vi "CC Script Parse Define Random Dithering.vi"(8 "error in (no error)":errorcluster, 9 "To Script?":bool, 10 "Dithering Offsets in":T1, 11 "DefineDithering Parameters":string="\"Rnadome Dither Mispeller\" Count=3,Radius=1.23") -> (0 "error out":errorcluster, 1 "Name":string, 2 "Dithering Offsets out":T1, 3 "Script out":string="ObjectName \"RA\":\"123.456\",\"DEC\":\"4546.54\"")   [LabVIEW 2020]
uses:
  <vilib>/regexp/Match Regular Expression.xnode
  typedefs/CC Dithering Offsets.ctl
  typedefs/CC Dithering.ctl
  typedefs/CC cluster Offset Dithering.ctl
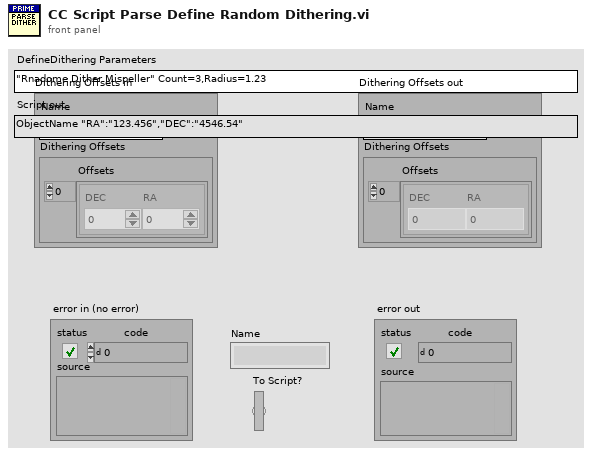
[diagram p1: front panel]
types:
  T1 = typedef "CC Dithering.ctl" = cluster{"Name":string, "Dithering Offsets":T2}
  T2 = typedef "CC cluster Offset Dithering.ctl" = cluster{"Offsets":T3[]}
  T3 = typedef "CC Dithering Offsets.ctl" = cluster{"DEC":dbl, "RA":dbl}
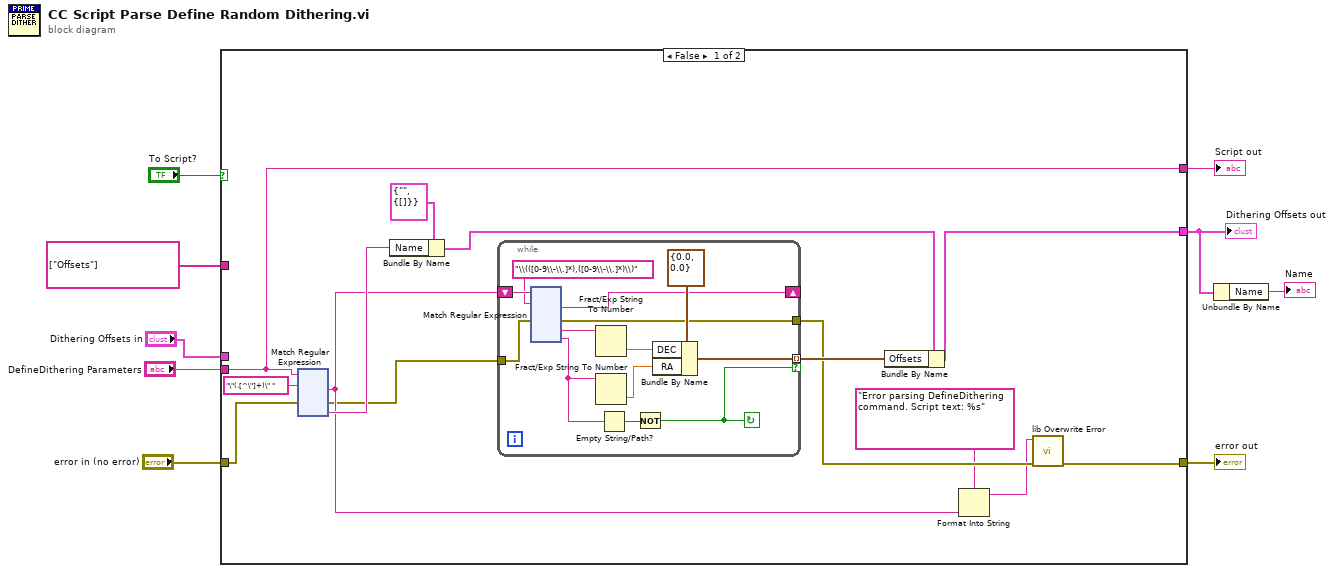
[diagram p0: block diagram]
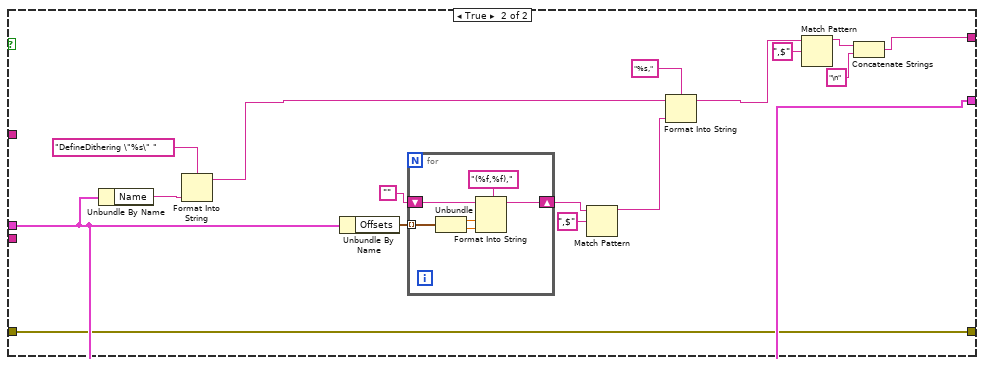
[diagram p2: hidden frame]
diagram:
  n1 = case shown="False" "To Script?" {
    tunnel: "DefineDithering Parameters" -> [w18 _]
    tunnel: string[] ["Offsets"] -> [_ _]
    tunnel: [w20 w278] -> w2
    tunnel: "error in (no error)" -> [w11 w276]
    tunnel: [w16 w276] -> w6
    tunnel: "Dithering Offsets in" -> [_ w278]
    tunnel: [w18 w277] -> w3
    frame False {
      n2 = xnode "Match Regular Expression"("input string"=w18, "regular expression"="\"(.[^\"]+)\" ", "error in"=w11) -> ("after match"=w13:string, "error out"=w10:errorcluster, "submatch 1"=w22:string)  [unwired: 3 in, 3 out]
      n3 = Bundle By Name(cluster=T1 {"Name"="", "Dithering Offsets"={"Offsets"=[]}} ("Dithering Offsets"), "Name"=w22) -> (w21:T1)
      n4 = while {
        shift-right: [w29] -> _
        shift-left: w13 -> [w36]
        tunnel: w10 -> [w34]
        tunnel: [w28] -> w17 mode=indexing if=w25
        tunnel: [w24] -> w15
        stop <- w25 continue-if-true
        n5 = xnode "Match Regular Expression"("input string"=w36, "regular expression"="\\(([0-9\\-\\.]*),([0-9\\-\\.]*)\\)", "error in"=w34) -> ("after match"=w29:string, "error out"=w24:errorcluster, "submatch 1"=w33:string, "submatch 2"=w27:string)  [unwired: 3 in, 3 out]
        n6 = Fract/Exp String To Number(string=w33) -> (number=w31:dbl)  [unwired: 3 in, 1 out]
        n7 = Fract/Exp String To Number(string=w27) -> (number=w30:dbl)  [unwired: 3 in, 1 out]
        n8 = Empty String/Path?(string/path=w27) -> (empty?=w26:bool)
        n9 = Not(x=w26) -> (.not. x?=w25:bool)
        n10 = Bundle By Name(cluster=T3 {"DEC"=0.0, "RA"=0.0} ("Dither Offsets"), "DEC"=w31, "RA"=w30) -> (w28:T3)
      }
      n11 = Bundle By Name(cluster=w21, "Offsets"=w17) -> (w20:T1)
      n12 = Format Into String(format string="Error parsing DefineDithering command. Script text: %s", w13) -> (resulting string=w12:string)  [unwired: 2 in, 1 out]
      n13 = call "lib Overwrite Error.vi"("error in (no error)"=w15, "Error Message"=w12) -> ("error out"=w16:errorcluster)  [unwired: 9 in]
    }
    frame True {
      n14 = Unbundle By Name(w278) -> ("Name"=w284:string)
      n15 = Format Into String(format string="DefineDithering \"%s\" ", w284) -> (resulting string=w283:string)  [unwired: 2 in, 1 out]
      n16 = Unbundle By Name(w278) -> ("Offsets"=w272:T3[])
      n17 = for {
        shift-right: [w289] -> w270
        shift-left: "" -> [w290]
        tunnel: w272 -> [w288] mode=indexing
        n18 = Unbundle(w288) -> ("DEC"=w286:dbl, "RA"=w287:dbl)
        n19 = Format Into String(format string="(%f,%f),", initial string=w290, w286, w287) -> (resulting string=w289:string)  [unwired: 1 in, 1 out]
      }
      n20 = Match Pattern(string=w270, regular expression=",$") -> (before substring=w274:string)  [unwired: 1 in, 3 out]
      n21 = Format Into String(format string="%s,", initial string=w283, w274) -> (resulting string=w282:string)  [unwired: 1 in, 1 out]
      n22 = Match Pattern(string=w282, regular expression=",$") -> (before substring=w280:string)  [unwired: 1 in, 3 out]
      n23 = Concatenate Strings(w280, "\n" ("string")) -> (w277:string)
    }
  }
  "error out" <- w6
  "Dithering Offsets out" <- w2
  "Script out" <- w3
  n24 = Unbundle By Name(w2) -> ("Name"=→"Name":string)
